vi "ReplyToOneGraph.vi"(7 "ServerActions":T1, 8 "error in (no error)":errorcluster, 9 "Graph name":string, 10 "data":variant, 11 "Gserver in":refnum<class "Gserver.lvclass">) -> (0 "error out":errorcluster, 3 "Gserver out":refnum<class "Gserver.lvclass">)   [LabVIEW 2020, in "Gserver.lvclass"]
doc: "Andre Koelewijn, 5 jan 2021\n\nSend a reply to one Gview Graph instance as identified by Graph name"
uses:
  Gserver.lvclass
  Gview/controls/Typedef_ServerActions.ctl
  Gserver.lvclass/Gserver.ctl
  Gview/controls/Typedef_Gserver-Replies.ctl
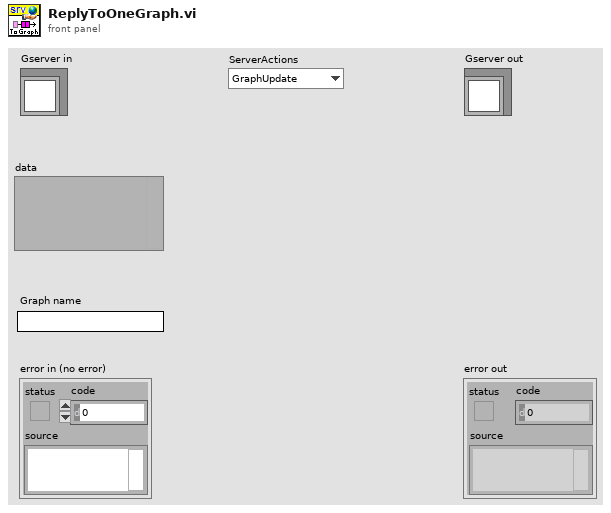
[diagram p1: front panel]
types:
  T1 = typedef "Typedef_ServerActions.ctl" = enum16{"GraphUpdate", "SendAllTags", "SendIniPath", "SetGeneralOptions", "EditTagsOpen", "EditTagsPresetSave", "EditTagsPresetLoad", "EditTagsClose", "NewTagSelection", "ExitGraph"}
  T2 = typedef "Typedef_Gserver-Replies.ctl" = cluster{"ServerActions":T1, "data":variant, "Source":string, "Time Stamp":timestamp}
  T3 = typedef "Gserver.lvclass/Typedef_Sgraph_Query.ctl" = cluster{"ViewportName":string, "Tags":string[], "Time-Start":timestamp, "Time-End":timestamp, "Pixels":i32, "Live":T4, "TimeSpan(sec)":dbl, "GViewer-Queue":refnum<queue>}
  T4 = typedef "Gviewer.lvclass/Typedef_Live.ctl" = enum16{"Live View", "Freeze"}
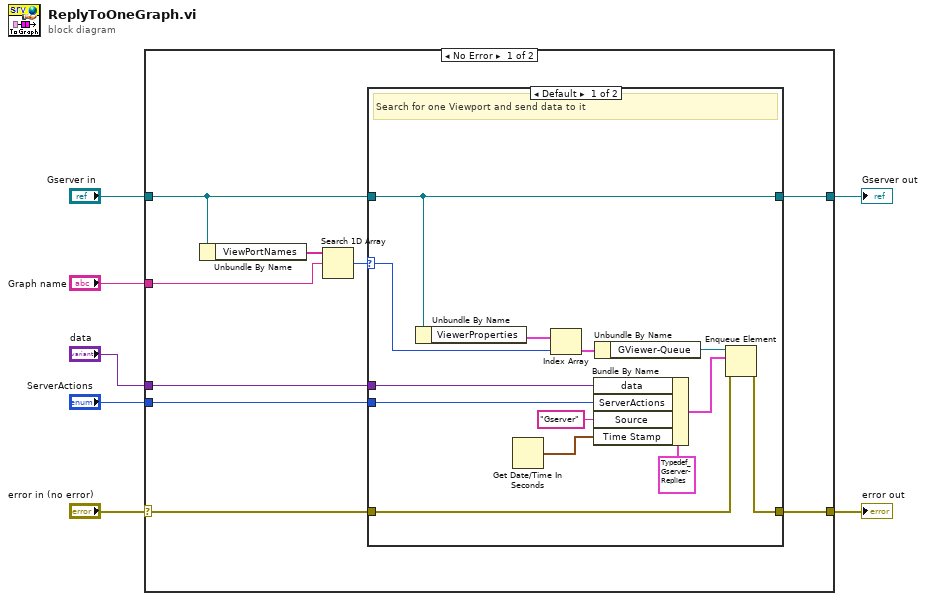
[diagram p0: block diagram]
diagram:
  n1 = case shown="No Error" "error in (no error)" {
    selector: "error in (no error)" -> [w13 w33]
    tunnel: [w12 w33] -> w6
    tunnel: [w9 w32] -> w4
    tunnel: "Gserver in" -> [w8 w32]
    tunnel: "Graph name" -> [w14 _]
    tunnel: "ServerActions" -> [w11 _]
    tunnel: "data" -> [w10 _]
    frame No Error {
      n2 = Unbundle By Name(w8) -> ("ViewPortNames"=w16:string[])
      n3 = Search 1D Array(1D array=w16, element=w14) -> (index of element=w15:i32)  [unwired: 1 in]
      n4 = case shown="Default" w15 {
        selector: w15 -> [w28 _]
        tunnel: w8 -> [w17 w31]
        tunnel: [w17 w31] -> w9
        tunnel: w13 -> [w21 w30]
        tunnel: [w20 w30] -> w12
        tunnel: w11 -> [w19 _]
        tunnel: w10 -> [w18 _]
        frame Default {
          # "Search for one Viewport and send data to it"
          n5 = Unbundle By Name(w17) -> ("ViewerProperties"=w29:T3[])
          n6 = Get Date/Time In Seconds() -> (seconds since 1Jan1904=w26:timestamp)
          n7 = Index Array(array=w29, index=w28) -> (element=w24:T3)
          n8 = Bundle By Name(cluster=T2 {"ServerActions"=enum."GraphUpdate", "data"=variant, "Source"="", "Time Stamp"=timestamp(0 s since 1904-01-01)} ("element"), "data"=w18, "ServerActions"=w19, "Source"="Gserver", "Time Stamp"=w26) -> (w22:T2)
          n9 = Unbundle By Name(w24) -> ("GViewer-Queue"=w27:refnum<queue>)
          n10 = Enqueue Element(queue=w27, element=w22, error in (no error)=w21) -> (error out=w20:errorcluster)  [unwired: 1 in, 2 out]
        }
        frame -1 {
          # "Viewport Graph not found"
        }
      }
    }
    frame Error {
    }
  }
  "error out" <- w6
  "Gserver out" <- w4
